vi "initROI.vi"(11 "Cam out":T2) -> (1 "Screen&Camera 2":T8, 2 "ROI info":T1, 3 "UserROI":T7)   [LabVIEW 2020]
uses:
  CamRoiTypDef.ctl
  ScreenCam2_TypDEf.ctl
  CamAndObj_TypDEf.ctl
  CamSettingSUB_TypDEf.ctl
  OnOffTypeDef.ctl
  userROI.ctl
  source/Device Drivers/shared/numericVariable_TypeDef.ctl
  ROIInfo_TypDef.ctl
  source/Device Drivers/BaseDriver/BaseDriver.lvclass
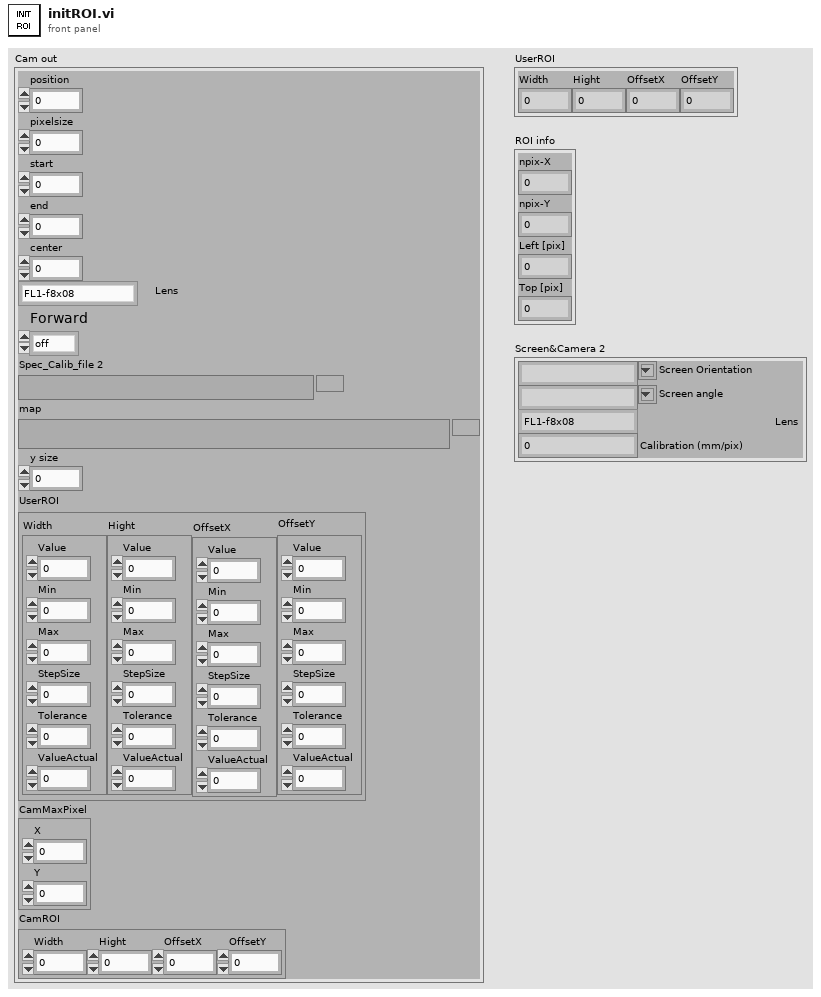
[diagram p1: front panel]
types:
  T1 = typedef "ROIInfo_TypDef.ctl" = cluster{"npix-X":i32, "npix-Y":i32, "Left [pix]":dbl, "Top [pix]":dbl}
  T2 = typedef "CamSettingSUB_TypDEf.ctl" = cluster{"position":dbl, "pixelsize":dbl, "start":dbl, "end":dbl, "center":dbl, "Lens":T3, "Forward":T4, "Spec_Calib_file 2":path, "map":path, "y size":i32, "UserROI":T5, "CamMaxPixel":cluster{"X":i32, "Y":i32}, "CamROI":T7}
  T3 = typedef "CamAndObj_TypDEf.ctl" = enum16{"FL1-f8x08", "FL1-f8x06", "FL1-f8", "ch300-f50", "FL2G-f8", "FL3M14-f8", "FL3M14-f8x08", "FL3M14-f8x08(2x2)"}
  T4 = typedef "OnOffTypeDef.ctl" = enum16{"off", "on"}
  T5 = typedef "userROI.ctl" = cluster{"Width":T6, "Hight":T6, "OffsetX":T6, "OffsetY":T6}
  T6 = typedef "BaseDriver.lvclass/numericVariable_TypeDef.ctl" = cluster{"Value":dbl, "Min":dbl, "Max":dbl, "StepSize":dbl, "Tolerance":dbl, "ValueActual":dbl}
  T7 = typedef "CamRoiTypDef.ctl" = cluster{"Width":dbl, "Hight":dbl, "OffsetX":dbl, "OffsetY":dbl}
  T8 = typedef "ScreenCam2_TypDEf.ctl" = cluster{"Screen Orientation":string, "Screen angle":string, "Lens":T3, "Calibration (mm/pix)":dbl}
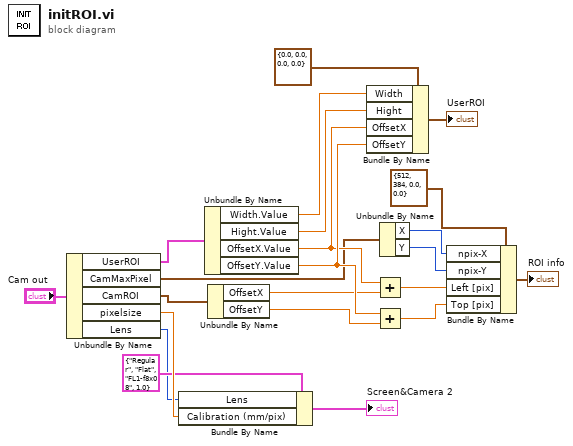
[diagram p0: block diagram]
diagram:
  n1 = Unbundle By Name("Cam out") -> ("UserROI"=w17:T5, "CamMaxPixel"=w7:cluster{"X":i32, "Y":i32}, "CamROI"=w10:T7, "pixelsize"=w14:dbl, "Lens"=w3:T3)
  n2 = Bundle By Name(cluster=T8 {"Screen Orientation"="Regular", "Screen angle"="Flat", "Lens"=enum."FL1-f8x08", "Calibration (mm/pix)"=1.0} ("Screen&Camera 2"), "Lens"=w3, "Calibration (mm/pix)"=w14) -> (→"Screen&Camera 2":T8)
  n3 = Unbundle By Name(w17) -> ("Width.Value"=w19:dbl, "Hight.Value"=w20:dbl, "OffsetX.Value"=w21:dbl, "OffsetY.Value"=w22:dbl)
  n4 = Unbundle By Name(w10) -> ("OffsetX"=w13:dbl, "OffsetY"=w11:dbl)
  n5 = Bundle By Name(cluster=T7 {"Width"=0.0, "Hight"=0.0, "OffsetX"=0.0, "OffsetY"=0.0} ("UserROI"), "Width"=w19, "Hight"=w20, "OffsetX"=w21, "OffsetY"=w22) -> (→"UserROI":T7)
  n6 = Add(x=w21, y=w13) -> (x+y=w15:dbl)
  n7 = Add(x=w22, y=w11) -> (x+y=w12:dbl)
  n8 = Unbundle By Name(w7) -> ("X"=w8:i32, "Y"=w9:i32)
  n9 = Bundle By Name(cluster=T1 {"npix-X"=512, "npix-Y"=384, "Left [pix]"=0.0, "Top [pix]"=0.0} ("ROI info"), "npix-X"=w8, "npix-Y"=w9, "Left [pix]"=w15, "Top [pix]"=w12) -> (→"ROI info":T1)
